vi "Handle Nested Error.vi"(8 "error in (no error)":errorcluster, 10 "Nested Error":errorcluster, 11 "Actor Nest in":refnum<class "Actor Nest.lvclass">) -> (0 "error out":errorcluster, 3 "Actor Nest out":refnum<class "Actor Nest.lvclass">)   [LabVIEW 2018, in "Actor Nest.lvlib" / "Actor Nest.lvclass"]
uses:
  Actor Nest.lvclass
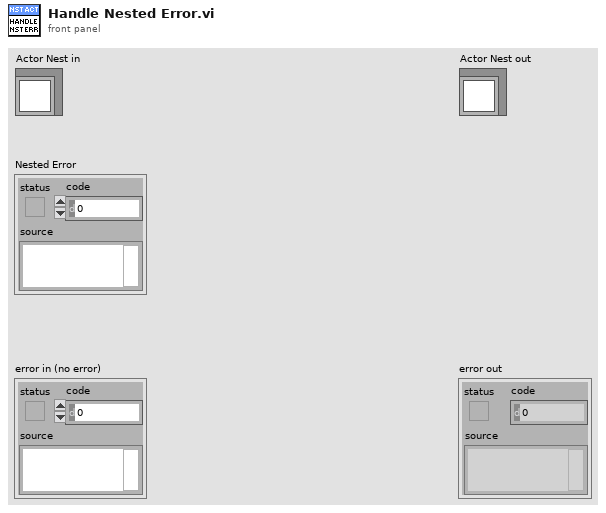
[diagram p1: front panel]
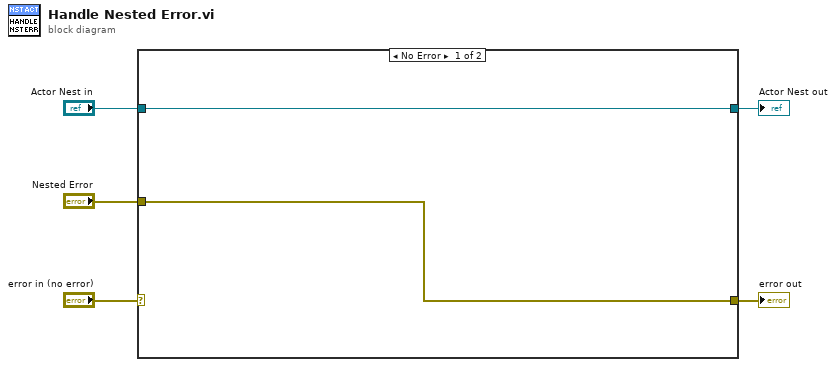
[diagram p0: block diagram]
diagram:
  n1 = case shown="No Error" "error in (no error)" {
    selector: "error in (no error)" -> [_ w9]
    tunnel: [w6 w9] -> w4
    tunnel: [w7 w8] -> w2
    tunnel: "Actor Nest in" -> [w7 w8]
    tunnel: "Nested Error" -> [w6 _]
    frame No Error {
    }
    frame Error {
    }
  }
  "error out" <- w4
  "Actor Nest out" <- w2
